vi "Tester.vi"() -> ()   [LabVIEW 2012]
uses:
  <instrlib>/Olympus IX BX Series/Olympus IX BX Series.lvlib
panel:
  out "number":dbl format="%#.3f"
  in  "Stop Motion":bool
  in  "Absolute (0.0 um)":dbl format="%.1f"
  in  "VISA Resource Name":refnum<visa-resource-name>="ASRL1"
  out "Result":string
  in  "Step (0.0 um)":dbl format="%.1f"
  in  "Direction (1: Down)":enum16{"Up", "Down", "Absolute"}(ring)=enum."Down"
  in  "Move":bool
  in  "stop":bool
  out "error out":errorcluster {"code" format="%.0x"}
  in  "ID Query? (F: No)":bool
  in  "Device Number (1)":i32=2
  in  "Serial Configuration":T1={"Baud Rate (19200)"=19200, "Flow Control (2: RTS/CTS)"=2, "Parity (2: Even)"=2, "Data Bits (8)"=8, "Stop Bits (20: 2.0)"=20} {"Stop Bits (20: 2.0)" items=["1.0"=10, "1.5"=15, "2.0"=20]; "Data Bits (8)" items=["7"=7, "8"=8]; "Parity (2: Even)" items=["None", "Odd", "Even", "Mark", "Space"]; "Flow Control (2: RTS/CTS)" items=["None"=0, "XON/XOFF"=1, "RTS/CTS"=2, "DTR/DSR"=4]; "Baud Rate (19200)" items=["300"=300, "600"=600, "1200"=1200, "2400"=2400, "4800"=4800, "9600"=9600, "19200"=19200]}
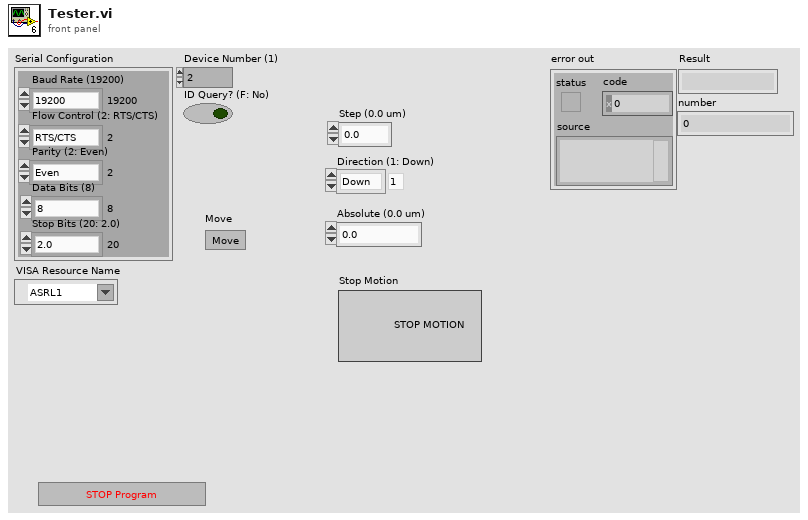
[diagram p1: front panel]
types:
  T1 = cluster{"Baud Rate (19200)":u32, "Flow Control (2: RTS/CTS)":u16, "Parity (2: Even)":u16, "Data Bits (8)":u16, "Stop Bits (20: 2.0)":u16}
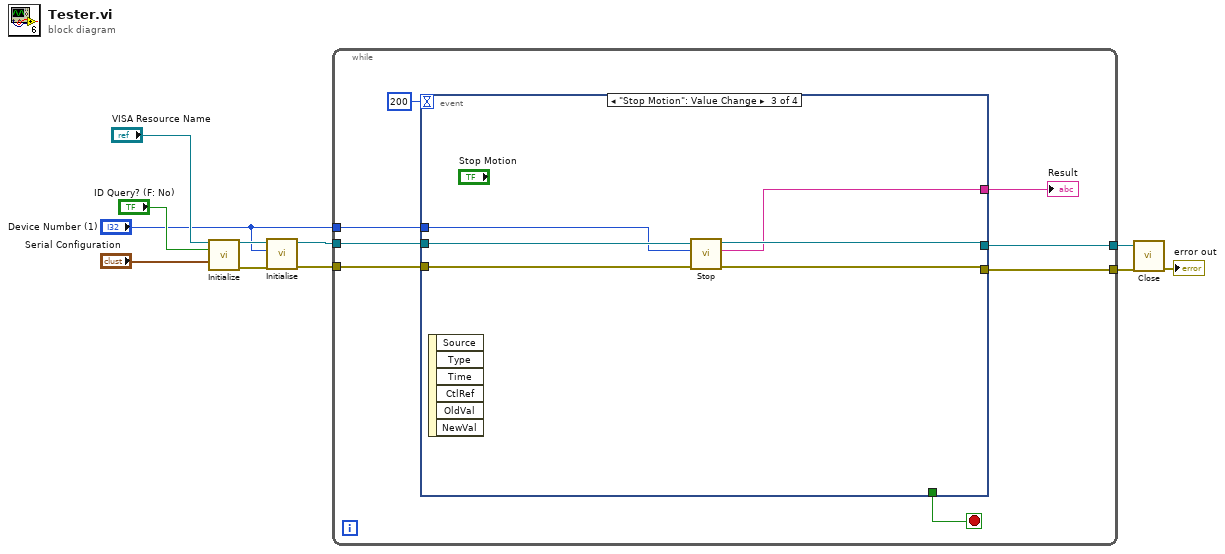
[diagram p0: block diagram]
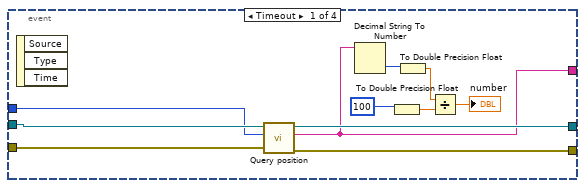
[diagram p2: hidden frame]
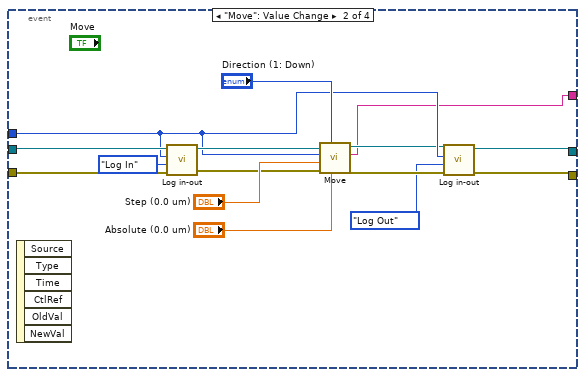
[diagram p3: hidden frame]
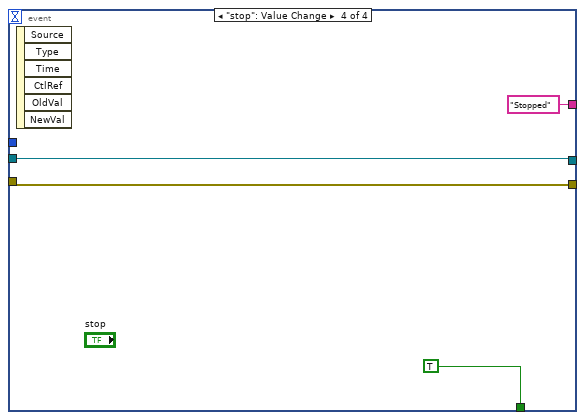
[diagram p4: hidden frame]
diagram:
  n1 = call <instrlib>:"Initialize.vi"("VISA Resource Name"="VISA Resource Name", "ID Query? (F: No)"="ID Query? (F: No)", "Serial Configuration"="Serial Configuration") -> ("VISA Resource Name Out"=w11:refnum<visa-resource-name>, "error out"=w10:errorcluster)  [unwired: 11 in]
  n2 = call "Initialise.vi"("error in (no error)"=w10, "Device Number (1)"="Device Number (1)", "VISA Resource Name"=w11) -> ("error out"=w6:errorcluster, "VISA Resource Name Out"=w7:refnum<visa-resource-name>)  [unwired: 6 in, 1 out]
  n3 = while {
    tunnel: w7 -> [w18]
    tunnel: w6 -> [w17]
    tunnel: "Device Number (1)" -> [w16]
    tunnel: [w15] -> w5
    tunnel: [w14] -> w4
    stop <- w13 stop-if-true
    n4 = event shown="[2] \"Stop Motion\": Value Change" {
      selector: _ -> [_ _ _ _]
      dyn-events: _ -> [_ _ _ _]
      timeout: 200 -> [_ _ _ _]
      tunnel: w18 -> [w30 w42 w50 w53]
      tunnel: w17 -> [w29 w43 w51 w52]
      tunnel: w16 -> [w28 w38 w46 _]
      tunnel: [w27 w35 w49 w53] -> w15
      tunnel: [w26 w34 w48 w52] -> w14
      tunnel: [_ _ _ TRUE] -> w13
      tunnel: [w25 w32 w47 "Stopped" ("Result")] -> w12
      event Timeout {
        n5 = event-data() -> ()  [unwired: 1 in, 3 out]
        n6 = call "Query position.vi"("error in (no error)"=w29, "Device Number (1)"=w28, "VISA Resource Name"=w30) -> ("error out"=w26:errorcluster, "Result"=w25:string, "VISA Resource Name Out"=w27:refnum<visa-resource-name>)  [unwired: 6 in]
        n7 = Decimal String To Number(string=w25) -> (number=w23:i32)  [unwired: 2 in, 1 out]
        n8 = To Double Precision Float(number=100 ("y")) -> (double precision float=w22:dbl)
        n9 = To Double Precision Float(number=w23) -> (double precision float=w20:dbl)
        n10 = Divide(x=w20, y=w22) -> (x/y=→"number":dbl)
      }
      event "Move": Value Change {
        n11 = event-data() -> ()  [unwired: 1 in, 6 out]
        n12 = call "Log in-out.vi"("error in (no error)"=w43, "Input"=enum16{"Log In", "Log Out"}."Log In", "Device Number (1)"=w38, "VISA Resource Name"=w42) -> ("error out"=w40:errorcluster, "VISA Resource Name Out"=w41:refnum<visa-resource-name>)  [unwired: 5 in, 1 out]
        n13 = call "Move.vi"("Absolute (0.0 um)"="Absolute (0.0 um)", "Direction (1: Down)"="Direction (1: Down)", "error in (no error)"=w40, "Step (0.0 um)"="Step (0.0 um)", "Device Number (1)"=w38, "VISA Resource Name"=w41) -> ("error out"=w39:errorcluster, "Result"=w32:string, "VISA Resource Name Out"=w33:refnum<visa-resource-name>)  [unwired: 3 in]
        n14 = call "Log in-out.vi"("error in (no error)"=w39, "Input"=enum16{"Log In", "Log Out"}."Log Out", "Device Number (1)"=w38, "VISA Resource Name"=w33) -> ("error out"=w34:errorcluster, "VISA Resource Name Out"=w35:refnum<visa-resource-name>)  [unwired: 5 in, 1 out]
      }
      event "Stop Motion": Value Change {
        n15 = event-data() -> ()  [unwired: 1 in, 6 out]
        n16 = call "Stop.vi"("error in (no error)"=w51, "Device Number (1)"=w46, "VISA Resource Name"=w50) -> ("error out"=w48:errorcluster, "Result"=w47:string, "VISA Resource Name Out"=w49:refnum<visa-resource-name>)  [unwired: 6 in]
      }
      event "stop": Value Change {
        n17 = event-data() -> ()  [unwired: 1 in, 6 out]
      }
    }
    "Result" <- w12
  }
  n18 = call <instrlib>:"Close.vi"("VISA Resource Name"=w5, "error in (no error)"=w4) -> ("error out"=→"error out":errorcluster)  [unwired: 13 in]
